vi "1C.3 SmallRCAct.vi"   [LabVIEW 2011]
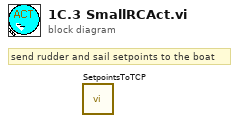
[diagram p0: block diagram]
diagram:
  # "send rudder and sail setpoints to the boat"
  n1 = call "SetpointsToTCP.vi"() -> ()  [unwired: 10 in, 2 out]
